vi "Read Elevator IDs from Config.vi"(8 "error in (no error)":errorcluster, 11 "Settings in":variant) -> (0 "error out":errorcluster, 2 "Elevator ID's":T1, 3 "Settings out":variant)   [LabVIEW 2019, in "Elevator.lvlib" / "Elevator.lvclass"]
doc: "This VI reads the elevator IDs from the variant settings connected to the subVI and returns the cluster with them populated."
uses:
  Elevator.lvclass
  Controls/Elevator IDs.ctl
  ca2d25cd-08f3-4a59-b13c-3eba346c896a.vi
  <vilib>/Utility/error.llb/Trim Whitespace.vi
  <vilib>/Utility/error.llb/Error Cluster From Error Code.vi
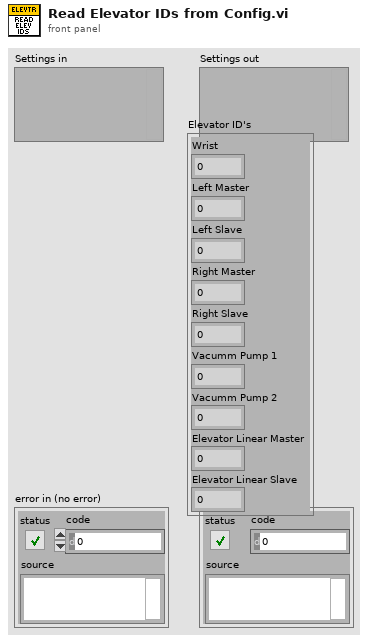
[diagram p1: front panel]
types:
  T1 = typedef "Elevator.lvlib/Elevator.lvclass/Elevator IDs.ctl" = cluster{"Wrist":u8, "Left Master":u8, "Left Slave":u8, "Right Master":u8, "Right Slave":u8, "Vacumm Pump 1":u8, "Vacumm Pump 2":u8, "Elevator Linear Master":u8, "Elevator Linear Slave":u8}
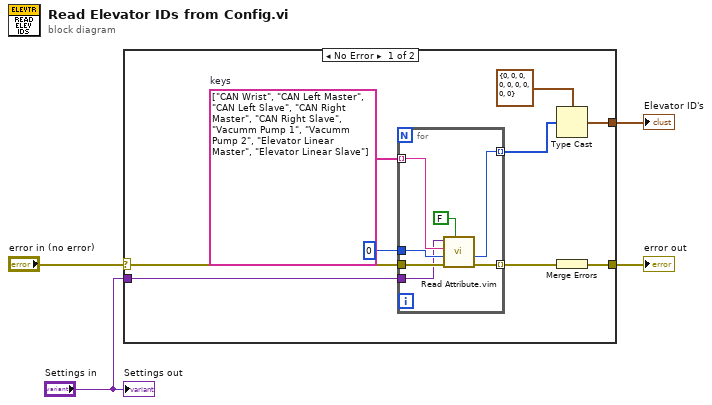
[diagram p0: block diagram]
diagram:
  n1 = case shown="No Error" "error in (no error)" {
    selector: "error in (no error)" -> [w13 w21]
    tunnel: [w9 w21] -> w4
    tunnel: "Settings in" -> [w5 _]
    tunnel: [w6 _] -> w2
    frame No Error {
      w11 = string[] ["CAN Wrist", "CAN Left Master", "CAN Left Slave", "CAN Right Master", "CAN Right Slave", "Vacumm Pump 1", "Vacumm Pump 2", "Elevator Linear Master", "Elevator Linear Slave"]  # keys
      n2 = for {
        tunnel: w11 -> [w20] mode=indexing
        tunnel: w13 -> [w18]
        tunnel: w5 -> [w16]
        tunnel: u8 0 -> [w17]
        tunnel: [w19] -> w8 mode=indexing
        tunnel: [w15] -> w10 mode=indexing
        n3 = call "Read Attribute.vim"("Error if not found (T)"=FALSE, "error in"=w18, "default value (data type)"=w17, "name"=w20, "variant in"=w16) -> ("error out"=w15:errorcluster, "value"=w19:u8)  [unwired: 3 in, 2 out]
      }
      n4 = Type Cast(type=T1 {"Wrist"=0, "Left Master"=0, "Left Slave"=0, "Right Master"=0, "Right Slave"=0, "Vacumm Pump 1"=0, "Vacumm Pump 2"=0, "Elevator Linear Master"=0, "Elevator Linear Slave"=0} ("Elevator ID's"), x=w8) -> (*(type *) &x=w6:T1)
      n5 = Merge Errors(w10) -> (w9:errorcluster)
    }
    frame Error {
    }
  }
  "error out" <- w4
  "Elevator ID's" <- w2
  "Settings out" <- "Settings in"
